vi "configureDigitalOutput.vi"(8 "error in (no error)":errorcluster, 9 "DigitalOutput":refnum<class "DigitalOutput.lvclass">, 10 "deviceName":string, 11 "AtomChipHWC in":refnum<class "AtomChipHWC.lvclass">) -> (0 "error out":errorcluster, 3 "AtomChipHWC out":refnum<class "AtomChipHWC.lvclass">)   [LabVIEW 2011, in "Hardware.lvlib" / "HWControllers.lvlib" / "AtomChipHWC.lvclass"]
doc: "Configure the digital output channels of a device"
uses:
  AtomChipHWC.lvclass
  Channels/Digital/DigitalOutput.lvclass
  AtomChipHWC.lvclass/AtomChipHWC.ctl
  HWController.lvclass
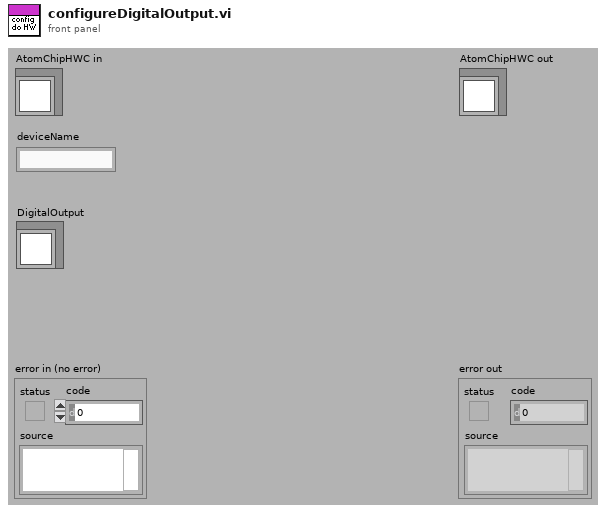
[diagram p1: front panel]
types:
  T1 = cluster{"Master Clock source":string, "Master Clock rate":dbl, "Start trigger line":string, "Scan rate":dbl, "Stop trigger line":string, "Sample Number":dbl}
  T2 = cluster{"Timestamps ms":dbl[], "DataPerChannel":dbl[][]}
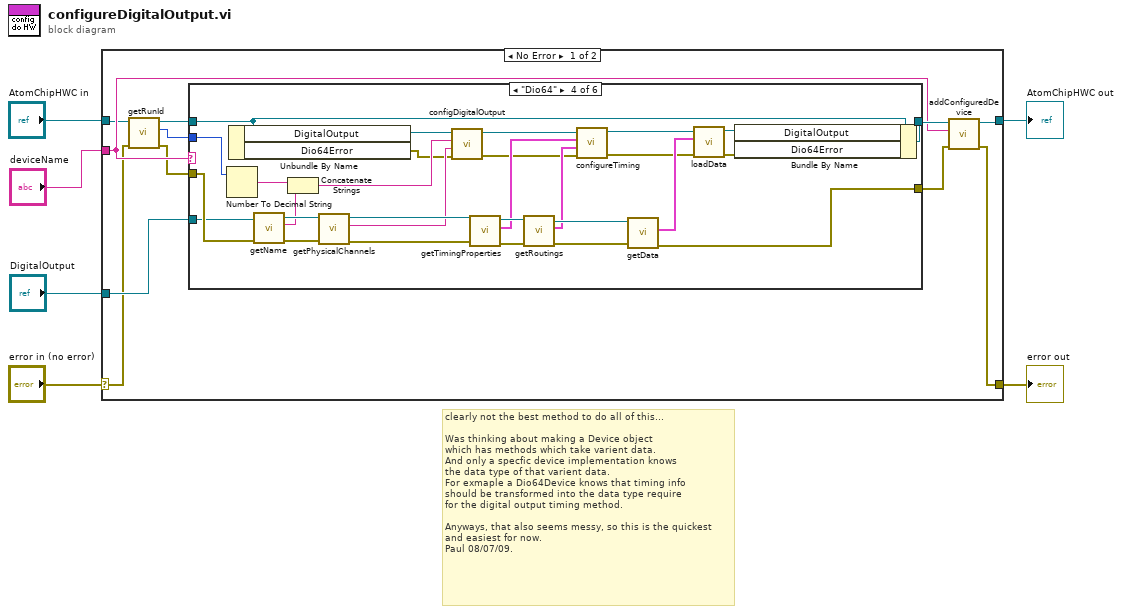
[diagram p0: block diagram]
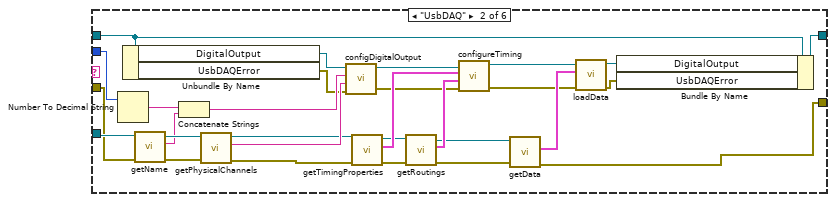
[diagram p3: hidden frame]
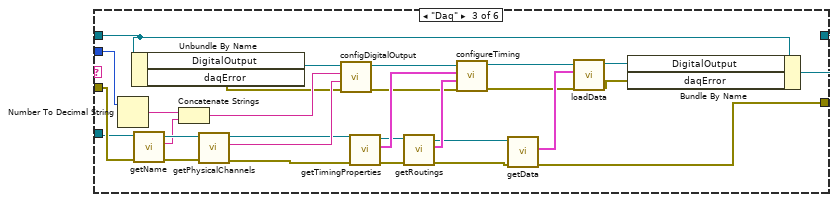
[diagram p4: hidden frame]
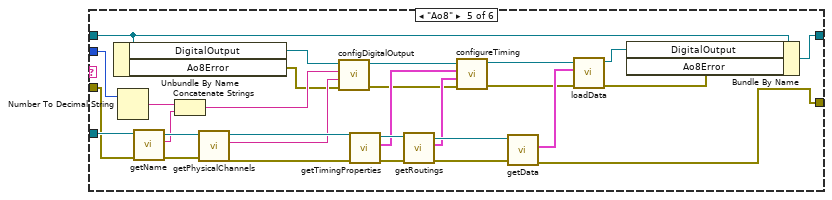
[diagram p5: hidden frame]
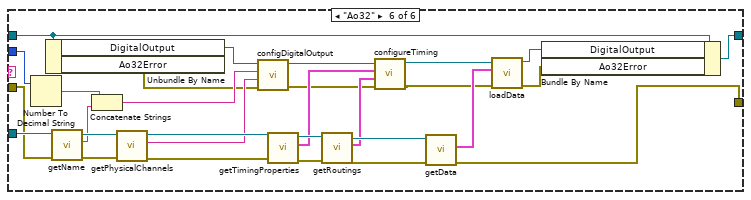
[diagram p6: hidden frame]
diagram:
  # "clearly not the best method to do all of this...\n \nWas thinking about making a Device object\nwhich has methods which take varient data.\nAnd only a specfic device implementation knows\nthe data type of that varient data. \nFor exmaple a Dio64Device knows that timing info\nshould be transformed into the data type require\nfor the digital output timing method.\n\nAnyways, that also seems messy, so this is the quickest\nand easiest for now.\nPaul 08/07/09."
  n1 = case shown="No Error" "error in (no error)" {
    selector: "error in (no error)" -> [w8 w166]
    tunnel: [w13 w166] -> w5
    tunnel: [w15 w165] -> w3
    tunnel: "AtomChipHWC in" -> [w11 w165]
    tunnel: "deviceName" -> [w12 _]
    tunnel: "DigitalOutput" -> [w17 _]
    frame No Error {
      n2 = call "getRunId.vi"("error in (no error)"=w8, "HWController in"=w11) -> ("error out"=w7:errorcluster, "Numeric"=w9:i32, "HWController out"=w10:refnum<class "AtomChipHWC.lvclass">)  [unwired: 7 in]
      n3 = case shown="\"Dio64\"" w12 {
        tunnel: w10 -> [w19 w34 w63 w93 w121 w149]
        tunnel: [w19 w33 w62 w92 w118 w148] -> w16
        tunnel: w7 -> [w18 w31 w61 w91 w119 w156]
        tunnel: [w18 w26 w50 w79 w109 w142] -> w14
        tunnel: w17 -> [_ w32 w60 w90 w120 w157]
        tunnel: w9 -> [_ w30 w58 w86 w116 w145]
        frame "No Hardware", Default {
        }
        frame "UsbDAQ" {
          n4 = Number To Decimal String(number=w30) -> (decimal integer string=w29:string)  [unwired: 1 in]
          n5 = Unbundle By Name(w34) -> ("DigitalOutput"=w42:refnum<class "DigitalOutput.lvclass">, "UsbDAQError"=w24:errorcluster)
          n6 = call-dynamic "getName.vi"("error in (no error)"=w31, "DigitalOutput.lvclass in"=w32) -> ("error out"=w37:errorcluster, "name"=w28:string, "DigitalOutput.lvclass out"=w36:refnum<class "DigitalOutput.lvclass">)  [unwired: 7 in]
          n7 = Concatenate Strings(w29, w28) -> (w27:string)
          n8 = call-dynamic "getPhysicalChannels.vi"("error in (no error)"=w37, "DigitalOutput.lvclass in"=w36) -> ("error out"=w23:errorcluster, "Physical Channels"=w43:string, "DigitalOutput.lvclass out"=w38:refnum<class "DigitalOutput.lvclass">)  [unwired: 7 in]
          n9 = call-dynamic "configDigitalOutput.vi"("error in (no error)"=w24, "Physical Channels"=w43, "name"=w27, "DigitalOutput in"=w42) -> ("error out"=w22:errorcluster, "DigitalOutput out"=w44:refnum<class "DigitalOutput.lvclass">)  [unwired: 6 in]
          n10 = call-dynamic "getTimingProperties.vi"("error in (no error)"=w23, "DigitalOutput.lvclass in"=w38) -> ("error out"=w40:errorcluster, "Timing"=w45:T1, "DigitalOutput.lvclass out"=w39:refnum<class "DigitalOutput.lvclass">)  [unwired: 7 in]
          n11 = call-dynamic "getRoutings.vi"("error in (no error)"=w40, "DigitalOutput.lvclass in"=w39) -> ("error out"=w21:errorcluster, "Routings"=w46:cluster{"Master Clock Route":string[]}, "DigitalOutput.lvclass out"=w41:refnum<class "DigitalOutput.lvclass">)  [unwired: 7 in]
          n12 = call-dynamic "configureTiming.vi"("error in (no error)"=w22, "Routings"=w46, "Timing"=w45, "DigitalOutput in"=w44) -> ("error out"=w25:errorcluster, "DigitalOutput out"=w35:refnum<class "DigitalOutput.lvclass">)  [unwired: 6 in]
          n13 = call-dynamic "getData.vi"("error in (no error)"=w21, "DigitalOutput.lvclass in"=w41) -> ("error out"=w26:errorcluster, "Data"=w47:T2)  [unwired: 7 in, 1 out]
          n14 = call-dynamic "loadData.vi"("error in (no error)"=w25, "Data"=w47, "DigitalOutput in"=w35) -> ("error out"=w20:errorcluster, "DigitalOutput out"=w48:refnum<class "DigitalOutput.lvclass">)  [unwired: 7 in]
          n15 = Bundle By Name(cluster=w34, "DigitalOutput"=w48, "UsbDAQError"=w20) -> (w33:refnum<class "AtomChipHWC.lvclass">)
        }
        frame "Daq" {
          n16 = Number To Decimal String(number=w58) -> (decimal integer string=w59:string)  [unwired: 1 in]
          n17 = Unbundle By Name(w63) -> ("DigitalOutput"=w71:refnum<class "DigitalOutput.lvclass">, "daqError"=w53:errorcluster)
          n18 = call-dynamic "getName.vi"("error in (no error)"=w61, "DigitalOutput.lvclass in"=w60) -> ("error out"=w66:errorcluster, "name"=w57:string, "DigitalOutput.lvclass out"=w65:refnum<class "DigitalOutput.lvclass">)  [unwired: 7 in]
          n19 = Concatenate Strings(w59, w57) -> (w56:string)
          n20 = call-dynamic "getPhysicalChannels.vi"("error in (no error)"=w66, "DigitalOutput.lvclass in"=w65) -> ("error out"=w55:errorcluster, "Physical Channels"=w72:string, "DigitalOutput.lvclass out"=w67:refnum<class "DigitalOutput.lvclass">)  [unwired: 7 in]
          n21 = call-dynamic "configDigitalOutput.vi"("error in (no error)"=w53, "Physical Channels"=w72, "name"=w56, "DigitalOutput in"=w71) -> ("error out"=w52:errorcluster, "DigitalOutput out"=w73:refnum<class "DigitalOutput.lvclass">)  [unwired: 6 in]
          n22 = call-dynamic "getTimingProperties.vi"("error in (no error)"=w55, "DigitalOutput.lvclass in"=w67) -> ("error out"=w69:errorcluster, "Timing"=w74:T1, "DigitalOutput.lvclass out"=w68:refnum<class "DigitalOutput.lvclass">)  [unwired: 7 in]
          n23 = call-dynamic "getRoutings.vi"("error in (no error)"=w69, "DigitalOutput.lvclass in"=w68) -> ("error out"=w54:errorcluster, "Routings"=w75:cluster{"Master Clock Route":string[]}, "DigitalOutput.lvclass out"=w70:refnum<class "DigitalOutput.lvclass">)  [unwired: 7 in]
          n24 = call-dynamic "configureTiming.vi"("error in (no error)"=w52, "Routings"=w75, "Timing"=w74, "DigitalOutput in"=w73) -> ("error out"=w51:errorcluster, "DigitalOutput out"=w64:refnum<class "DigitalOutput.lvclass">)  [unwired: 6 in]
          n25 = call-dynamic "getData.vi"("error in (no error)"=w54, "DigitalOutput.lvclass in"=w70) -> ("error out"=w50:errorcluster, "Data"=w76:T2)  [unwired: 7 in, 1 out]
          n26 = call-dynamic "loadData.vi"("error in (no error)"=w51, "Data"=w76, "DigitalOutput in"=w64) -> ("error out"=w49:errorcluster, "DigitalOutput out"=w77:refnum<class "DigitalOutput.lvclass">)  [unwired: 7 in]
          n27 = Bundle By Name(cluster=w63, "DigitalOutput"=w77, "daqError"=w49) -> (w62:refnum<class "AtomChipHWC.lvclass">)
        }
        frame "Dio64" {
          n28 = Number To Decimal String(number=w86) -> (decimal integer string=w89:string)  [unwired: 1 in]
          n29 = Unbundle By Name(w93) -> ("DigitalOutput"=w99:refnum<class "DigitalOutput.lvclass">, "Dio64Error"=w84:errorcluster)
          n30 = call-dynamic "getName.vi"("error in (no error)"=w91, "DigitalOutput.lvclass in"=w90) -> ("error out"=w104:errorcluster, "name"=w88:string, "DigitalOutput.lvclass out"=w105:refnum<class "DigitalOutput.lvclass">)  [unwired: 7 in]
          n31 = Concatenate Strings(w89, w88) -> (w87:string)
          n32 = call-dynamic "getPhysicalChannels.vi"("error in (no error)"=w104, "DigitalOutput.lvclass in"=w105) -> ("error out"=w83:errorcluster, "Physical Channels"=w98:string, "DigitalOutput.lvclass out"=w103:refnum<class "DigitalOutput.lvclass">)  [unwired: 7 in]
          n33 = call-dynamic "configDigitalOutput.vi"("error in (no error)"=w84, "Physical Channels"=w98, "name"=w87, "DigitalOutput in"=w99) -> ("error out"=w82:errorcluster, "DigitalOutput out"=w97:refnum<class "DigitalOutput.lvclass">)  [unwired: 6 in]
          n34 = call-dynamic "getTimingProperties.vi"("error in (no error)"=w83, "DigitalOutput.lvclass in"=w103) -> ("error out"=w101:errorcluster, "Timing"=w85:T1, "DigitalOutput.lvclass out"=w102:refnum<class "DigitalOutput.lvclass">)  [unwired: 7 in]
          n35 = call-dynamic "getRoutings.vi"("error in (no error)"=w101, "DigitalOutput.lvclass in"=w102) -> ("error out"=w80:errorcluster, "Routings"=w96:cluster{"Master Clock Route":string[]}, "DigitalOutput.lvclass out"=w100:refnum<class "DigitalOutput.lvclass">)  [unwired: 7 in]
          n36 = call-dynamic "configureTiming.vi"("error in (no error)"=w82, "Routings"=w96, "Timing"=w85, "DigitalOutput in"=w97) -> ("error out"=w81:errorcluster, "DigitalOutput out"=w106:refnum<class "DigitalOutput.lvclass">)  [unwired: 6 in]
          n37 = call-dynamic "getData.vi"("error in (no error)"=w80, "DigitalOutput.lvclass in"=w100) -> ("error out"=w79:errorcluster, "Data"=w95:T2)  [unwired: 7 in, 1 out]
          n38 = call-dynamic "loadData.vi"("error in (no error)"=w81, "Data"=w95, "DigitalOutput in"=w106) -> ("error out"=w78:errorcluster, "DigitalOutput out"=w94:refnum<class "DigitalOutput.lvclass">)  [unwired: 7 in]
          n39 = Bundle By Name(cluster=w93, "DigitalOutput"=w94, "Dio64Error"=w78) -> (w92:refnum<class "AtomChipHWC.lvclass">)
        }
        frame "Ao8" {
          n40 = Unbundle By Name(w121) -> ("DigitalOutput"=w128:refnum<class "DigitalOutput.lvclass">, "Ao8Error"=w107:errorcluster)
          n41 = Number To Decimal String(number=w116) -> (decimal integer string=w117:string)  [unwired: 1 in]
          n42 = call-dynamic "getName.vi"("error in (no error)"=w119, "DigitalOutput.lvclass in"=w120) -> ("error out"=w133:errorcluster, "name"=w115:string, "DigitalOutput.lvclass out"=w134:refnum<class "DigitalOutput.lvclass">)  [unwired: 7 in]
          n43 = Concatenate Strings(w117, w115) -> (w114:string)
          n44 = call-dynamic "getPhysicalChannels.vi"("error in (no error)"=w133, "DigitalOutput.lvclass in"=w134) -> ("error out"=w111:errorcluster, "Physical Channels"=w127:string, "DigitalOutput.lvclass out"=w132:refnum<class "DigitalOutput.lvclass">)  [unwired: 7 in]
          n45 = call-dynamic "configDigitalOutput.vi"("error in (no error)"=w107, "Physical Channels"=w127, "name"=w114, "DigitalOutput in"=w128) -> ("error out"=w112:errorcluster, "DigitalOutput out"=w126:refnum<class "DigitalOutput.lvclass">)  [unwired: 6 in]
          n46 = call-dynamic "getTimingProperties.vi"("error in (no error)"=w111, "DigitalOutput.lvclass in"=w132) -> ("error out"=w130:errorcluster, "Timing"=w125:T1, "DigitalOutput.lvclass out"=w131:refnum<class "DigitalOutput.lvclass">)  [unwired: 7 in]
          n47 = call-dynamic "getRoutings.vi"("error in (no error)"=w130, "DigitalOutput.lvclass in"=w131) -> ("error out"=w110:errorcluster, "Routings"=w124:cluster{"Master Clock Route":string[]}, "DigitalOutput.lvclass out"=w129:refnum<class "DigitalOutput.lvclass">)  [unwired: 7 in]
          n48 = call-dynamic "configureTiming.vi"("error in (no error)"=w112, "Routings"=w124, "Timing"=w125, "DigitalOutput in"=w126) -> ("error out"=w113:errorcluster, "DigitalOutput out"=w135:refnum<class "DigitalOutput.lvclass">)  [unwired: 6 in]
          n49 = call-dynamic "getData.vi"("error in (no error)"=w110, "DigitalOutput.lvclass in"=w129) -> ("error out"=w109:errorcluster, "Data"=w123:T2)  [unwired: 7 in, 1 out]
          n50 = call-dynamic "loadData.vi"("error in (no error)"=w113, "Data"=w123, "DigitalOutput in"=w135) -> ("error out"=w108:errorcluster, "DigitalOutput out"=w122:refnum<class "DigitalOutput.lvclass">)  [unwired: 7 in]
          n51 = Bundle By Name(cluster=w121, "DigitalOutput"=w122, "Ao8Error"=w108) -> (w118:refnum<class "AtomChipHWC.lvclass">)
        }
        frame "Ao32" {
          n52 = Number To Decimal String(number=w145) -> (decimal integer string=w146:string)  [unwired: 1 in]
          n53 = Unbundle By Name(w149) -> ("DigitalOutput"=w155:refnum<class "DigitalOutput.lvclass">, "Ao32Error"=w139:errorcluster)
          n54 = call-dynamic "getName.vi"("error in (no error)"=w156, "DigitalOutput.lvclass in"=w157) -> ("error out"=w162:errorcluster, "name"=w144:string, "DigitalOutput.lvclass out"=w163:refnum<class "DigitalOutput.lvclass">)  [unwired: 7 in]
          n55 = Concatenate Strings(w146, w144) -> (w140:string)
          n56 = call-dynamic "getPhysicalChannels.vi"("error in (no error)"=w162, "DigitalOutput.lvclass in"=w163) -> ("error out"=w143:errorcluster, "Physical Channels"=w154:string, "DigitalOutput.lvclass out"=w161:refnum<class "DigitalOutput.lvclass">)  [unwired: 7 in]
          n57 = call-dynamic "configDigitalOutput.vi"("error in (no error)"=w139, "Physical Channels"=w154, "name"=w140, "DigitalOutput in"=w155) -> ("error out"=w136:errorcluster, "DigitalOutput out"=w153:refnum<class "DigitalOutput.lvclass">)  [unwired: 6 in]
          n58 = call-dynamic "getTimingProperties.vi"("error in (no error)"=w143, "DigitalOutput.lvclass in"=w161) -> ("error out"=w159:errorcluster, "Timing"=w152:T1, "DigitalOutput.lvclass out"=w160:refnum<class "DigitalOutput.lvclass">)  [unwired: 7 in]
          n59 = call-dynamic "getRoutings.vi"("error in (no error)"=w159, "DigitalOutput.lvclass in"=w160) -> ("error out"=w141:errorcluster, "Routings"=w151:cluster{"Master Clock Route":string[]}, "DigitalOutput.lvclass out"=w158:refnum<class "DigitalOutput.lvclass">)  [unwired: 7 in]
          n60 = call-dynamic "configureTiming.vi"("error in (no error)"=w136, "Routings"=w151, "Timing"=w152, "DigitalOutput in"=w153) -> ("error out"=w137:errorcluster, "DigitalOutput out"=w164:refnum<class "DigitalOutput.lvclass">)  [unwired: 6 in]
          n61 = call-dynamic "getData.vi"("error in (no error)"=w141, "DigitalOutput.lvclass in"=w158) -> ("error out"=w142:errorcluster, "Data"=w150:T2)  [unwired: 7 in, 1 out]
          n62 = call-dynamic "loadData.vi"("error in (no error)"=w137, "Data"=w150, "DigitalOutput in"=w164) -> ("error out"=w138:errorcluster, "DigitalOutput out"=w147:refnum<class "DigitalOutput.lvclass">)  [unwired: 7 in]
          n63 = Bundle By Name(cluster=w149, "DigitalOutput"=w147, "Ao32Error"=w138) -> (w148:refnum<class "AtomChipHWC.lvclass">)
        }
      }
      n64 = call "addConfiguredDevice.vi"("error in (no error)"=w14, "deviceName"=w12, "HWController in"=w16) -> ("error out"=w13:errorcluster, "HWController out"=w15:refnum<class "AtomChipHWC.lvclass">)  [unwired: 7 in]
    }
    frame Error {
    }
  }
  "error out" <- w5
  "AtomChipHWC out" <- w3
